vi "decodeState.vi"(8 "error in (no error)":errorcluster, 10 "Data":i16[](array[numeric]), 11 "ISA010 in":refnum<class "ISA010.lvclass">) -> (0 "error out":errorcluster, 2 "JSON string":string, 3 "ISA010 out":refnum<class "ISA010.lvclass">)   [LabVIEW 2017, in "ISA010.lvlib" / "ISA010.lvclass"]
uses:
  ISA010.lvclass
  Parameters.ctl
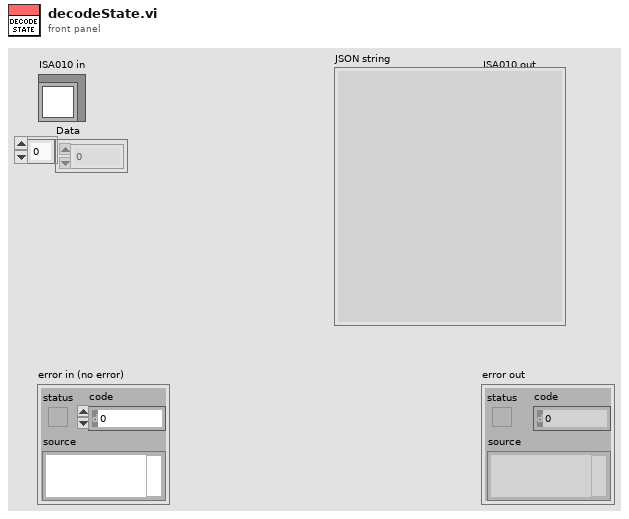
[diagram p1: front panel]
types:
  T1 = typedef "ISA010.lvlib/ISA010.lvclass/Parameters.ctl" = cluster{"Firmware":i16, "Outputs":i16, "Inputs":i16, "Uin":dbl, "PWM":i16, "Imp":i16, "Phat":i16, "DipSwitch":i16, "LockoutCode":i16, "Phase":i16, "PI2C":i16, "Texh":dbl, "ErrorCode":i16, "Vcc":i16, "Puart":i16, "dP":dbl, "Wejscia":cluster{"V1":bool, "V2":bool, "failure":bool, "DKG Power":bool}}
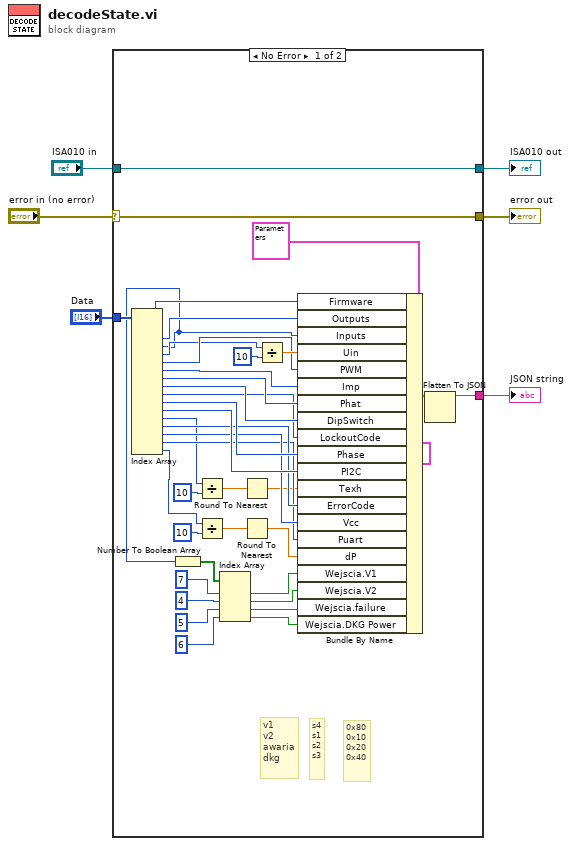
[diagram p0: block diagram]
diagram:
  n1 = case shown="No Error" "error in (no error)" {
    selector: "error in (no error)" -> [w44 w47]
    tunnel: [w44 w47] -> w5
    tunnel: [w45 w46] -> w3
    tunnel: "ISA010 in" -> [w45 w46]
    tunnel: "Data" -> [w43 _]
    tunnel: [w36 _] -> w1
    frame No Error {
      # "v1\nv2\nawaria\ndkg"
      # "0x80\n0x10\n0x20\n0x40"
      # "s4\ns1\ns2\ns3"
      n2 = Index Array(array=w43) -> (element #1=w42:i16, element #2=w41:i16, element #3=w7:i16, element #4=w17:i16, element #5=w34:i16, element #6=w33:i16, element #7=w32:i16, element #8=w31:i16, element #9=w30:i16, element #10=w29:i16, element #11=w28:i16, element #12=w22:i16, element #13=w27:i16, element #14=w26:i16, element #15=w25:i16, element #16=w24:i16)  [unwired: 16 in]
      n3 = Number To Boolean Array(number=w7) -> (Boolean array=w16:bool[])
      n4 = Divide(x=w22, y=i16 10) -> (x/y=w19:dbl)
      n5 = Divide(x=w24, y=i16 10) -> (x/y=w21:dbl)
      n6 = Index Array(array=w16, index #1=7 ("index"), index #2=4 ("index"), index #3=5 ("index"), index #4=6 ("index")) -> (element #1=w11:bool, element #2=w10:bool, element #3=w9:bool, element #4=w8:bool)
      n7 = Round To Nearest(number=w19) -> (nearest integer value=w18:dbl)
      n8 = Round To Nearest(number=w21) -> (nearest integer value=w20:dbl)
      n9 = Divide(x=w17, y=i16 10) -> (x/y=w39:dbl)
      n10 = Bundle By Name(cluster=T1 {"Firmware"=0, "Outputs"=0, "Inputs"=0, "Uin"=0.0, "PWM"=0, "Imp"=0, "Phat"=0, "DipSwitch"=0, "LockoutCode"=0, "Phase"=0, "PI2C"=0, "Texh"=0.0, "ErrorCode"=0, "Vcc"=0, "Puart"=0, "dP"=0.0, "Wejscia"={"V1"=FALSE, "V2"=FALSE, "failure"=FALSE, "DKG Power"=FALSE}} ("input cluster"), "Firmware"=w42, "Outputs"=w41, "Inputs"=w7, "Uin"=w39, "PWM"=w34, "Imp"=w33, "Phat"=w32, "DipSwitch"=w31, "LockoutCode"=w30, "Phase"=w29, "PI2C"=w28, "Texh"=w18, "ErrorCode"=w27, "Vcc"=w26, "Puart"=w25, "dP"=w20, "Wejscia.V1"=w11, "Wejscia.V2"=w10, "Wejscia.failure"=w9, "Wejscia.DKG Power"=w8) -> (w37:T1)
      n11 = Flatten To JSON(anything=w37) -> (JSON string=w36:string)  [unwired: 2 in, 1 out]
    }
    frame Error {
    }
  }
  "error out" <- w5
  "ISA010 out" <- w3
  "JSON string" <- w1
